vi "Kinematika.vi"() -> ()   [LabVIEW 2011]
uses:
  <vilib>/imath/engines/lvmath2/RunTimeEngine/ErrorHandling/NIMS_Finalize Error.vi
  <vilib>/imath/engines/lvmath2/RunTimeEngine/BuiltInFunctions/deg_to_rad/NIMS_deg_to_rad.vi
  <instcachedir>/0/NIMS_deg_to_rad_4A81D684CE8D4DD79924F5AB74D756E1.lvgen/NIMS_deg_to_rad_4A81D684CE8D4DD79924F5AB74D756E1_001.vi
  <vilib>/imath/engines/lvmath2/RunTimeEngine/NodeEndStatement/NIMS_NodeEndStatement_Output.vi
  <instcachedir>/0/NIMS_NodeEndStatement_Output_53EC0D466D134D7ABD903AC30B43404B.lvgen/NIMS_NodeEndStatement_Output_53EC0D466D134D7ABD903AC30B43404B_001.vi
  <instcachedir>/0/NIMS_NodeEndStatement_Output_53EC0D466D134D7ABD903AC30B43404B.lvgen/NIMS_NodeEndStatement_Output_53EC0D466D134D7ABD903AC30B43404B_012.vi
  <vilib>/imath/engines/lvmath2/RunTimeSupport/NIMS_Complex To Real.vi
  <instcachedir>/0/NIMS_Complex To Real_C6C689ECDA084B0290AC275552CC3682.lvgen/NIMS_Complex To Real_C6C689ECDA084B0290AC275552CC3682_001.vi
  <vilib>/imath/engines/lvmath2/RunTimeEngine/BuiltInFunctions/rad_to_deg/NIMS_rad_to_deg.vi
  <instcachedir>/0/NIMS_rad_to_deg_A39AFCDDC8C049FCADAAB7FC30B9F5AA.lvgen/NIMS_rad_to_deg_A39AFCDDC8C049FCADAAB7FC30B9F5AA_001.vi
  <vilib>/imathl/engines/lvmath/Functions/Error Handling/Create Error.vi
  <vilib>/imath/engines/lvmath2/RunTimeEngine/BuiltInFunctions/abs/NIMS_abs(signed).vi
  <instcachedir>/0/NIMS_abs(signed)_C4FCB8E6058B49B797C7C8D53CA5F6EC.lvgen/NIMS_abs(signed)_C4FCB8E6058B49B797C7C8D53CA5F6EC_002.vi
  <vilib>/imath/engines/lvmath2/RunTimeEngine/BuiltInFunctions/acos/NIMS_acos(C).vi
  <instcachedir>/0/NIMS_acos(C)_7CE2F6FACE8F41D2AB6320A13102A19C.lvgen/NIMS_acos(C)_7CE2F6FACE8F41D2AB6320A13102A19C_001.vi
  <vilib>/Instr/_visa.llb/VISA Configure Serial Port (Instr).vi
panel:
  in  "MOVE":bool
  in  "buffer":string
  in  "buffer":string
  out "PWM Values":T1
  in  "VISA NAME":refnum<visa-resource-name>="COM24"
  in  "STOP":bool
  in  "Dimensi Lengan Robot":cluster{"l1":dbl, "l2":dbl, "l3":dbl, "l4":dbl}={"l1"=75.0, "l2"=95.0, "l3"=95.0, "l4"=107.0} caption="Arm Dimensiions 2"
  out "TOP VIEW ROBOT":cluster{"Y":dbl[], "Y":dbl[]}[](graph)
  out "SIDE VIEW ROBOT":cluster{"Y":dbl[], "Y":dbl[]}[](graph)
  in  "Kinematik Maju / Balik":enum32{"Kinematika Maju", "Kinematika Balik"}(tab)
  out "Koordinat Akhir (KM)":cluster{"X":dbl, "Y":dbl, "Z":dbl}
  in  "BASE":dbl(knob) scale=-90.0..90.0
  in  "SHOULDER":dbl(knob)=30.0 scale=0.0..135.0
  in  "ELBOW":dbl(knob)=150.0 scale=90.0..270.0
  in  "WRIST":dbl(knob)=150.0 scale=90.0..270.0
  in  "ELBOW CONFIG":bool
  in  "Koordinat Z":dbl(slide)=75.0 scale=0.0..300.0
  in  "Koordinat Y":dbl(slide) scale=-135.0..135.0
  in  "Koordinat X":dbl(slide)=297.0 scale=0.0..300.0
  out "Sudut Persendian (KB)":cluster{"q1":dbl, "q2":dbl, "q3":dbl, "q4":dbl}
  in  "theta":dbl(knob) scale=0.0..90.0
  # "Percobaan kinematika maju ini didasarkan pada konfigurasi robot berlengan yang terintegrasi dengan sistem. \nRobot yang digunakan merupakan robot revolute yang memiliki 4 DOF ditambah satu gripper.\nRentang sudut yang diperbolehkan juga berdasarkan karakteristik penggerak robot\n\nParameter D-H  robot dapat dilihat pada tabel disamping."
  # "Percobaan kinematika balik ini merupakan perhitungan balik dari \npercobaan kinematika maju pada tab sebelumnya.\nsolusi kinematika balik yang beragam ditampilkan pada simulasi\ndengan memilih konfigurasi elbow up atau elbow down \nnamun robot berlengan yang terintegrasi dengan sistem hanya \nmenggunakan konfigurasi elbow up"
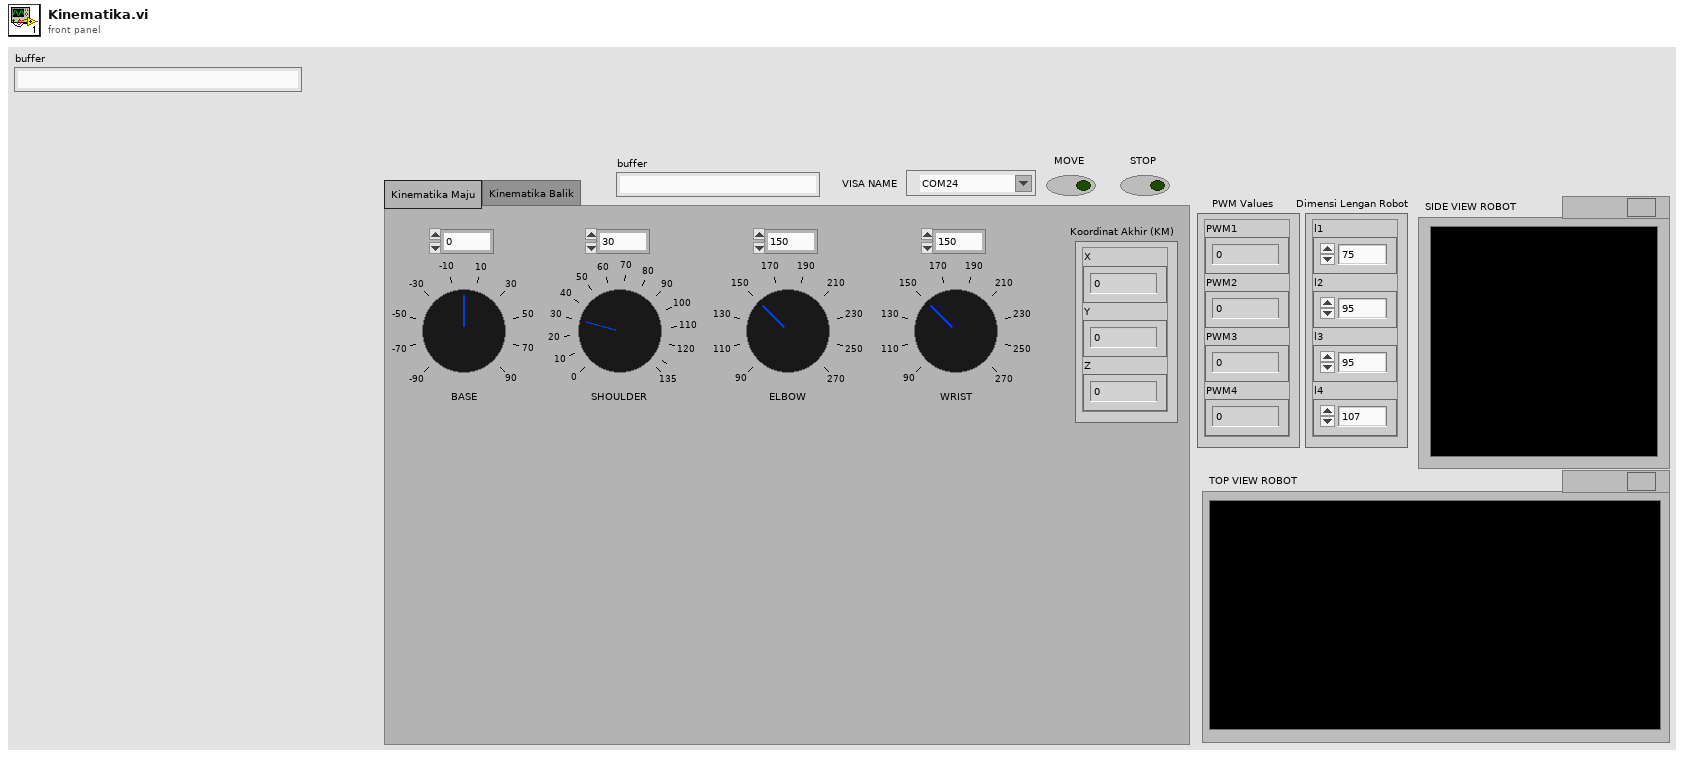
[diagram p1: front panel]
types:
  T1 = cluster{"PWM1":u32, "PWM2":u32, "PWM3":u32, "PWM4":u32}
  T2 = cluster{"PW1":u32, "PW2":u32, "PW3":u32, "PW4":u32}
  T3 = cluster{"Theta0":dbl, "Theta1":dbl, "Theta2":dbl}
  T4 = cluster{"Theta0":dbl, "Theta1":dbl, "Theta2":dbl, "Theta3":dbl}
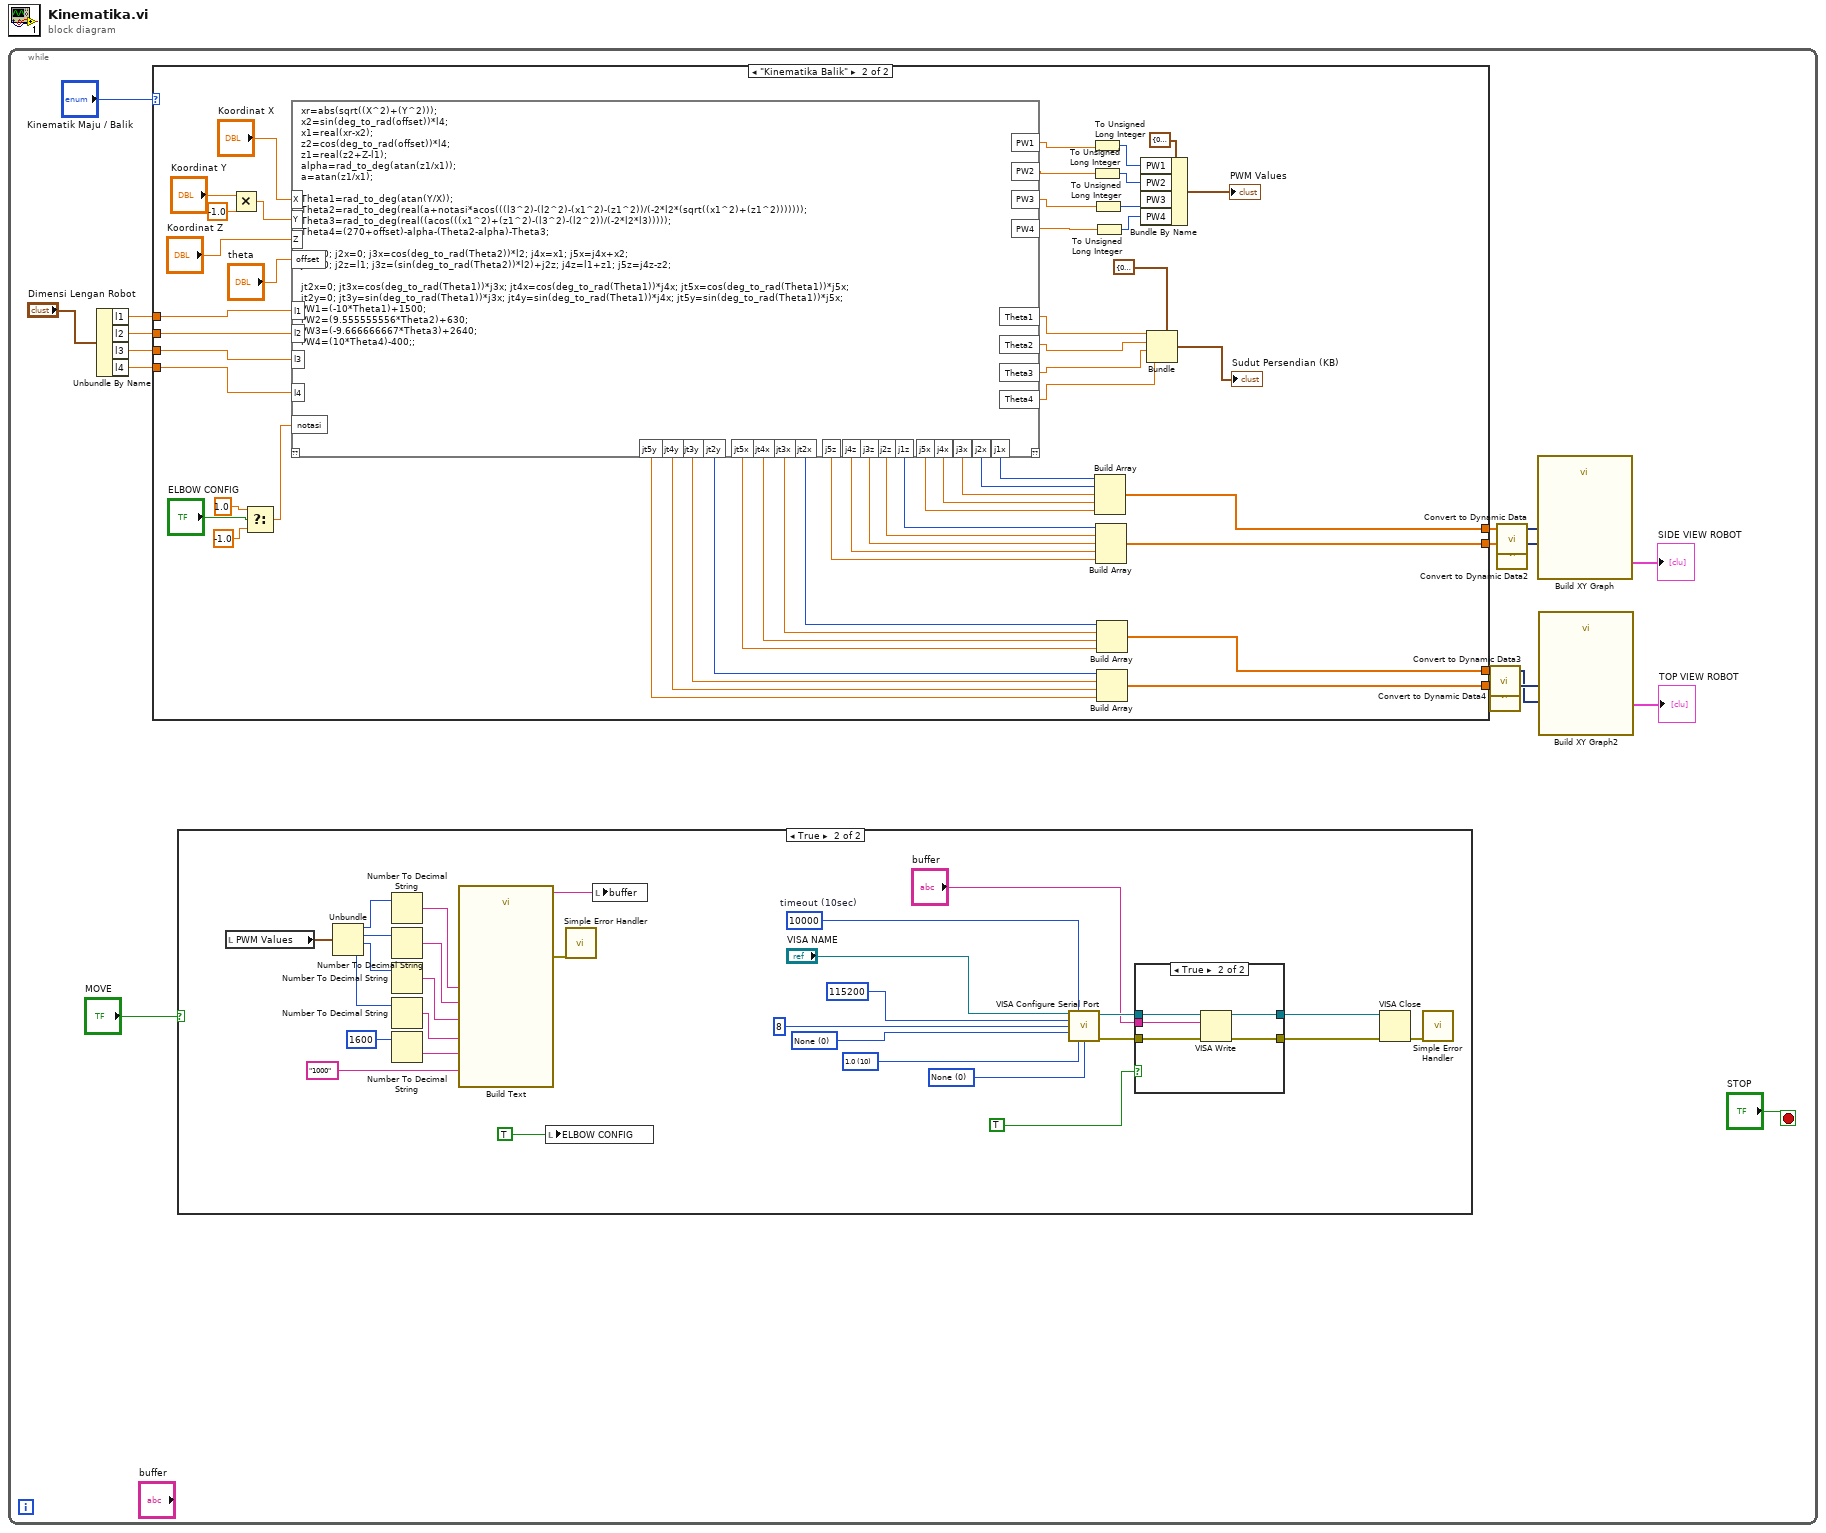
[diagram p0: block diagram]
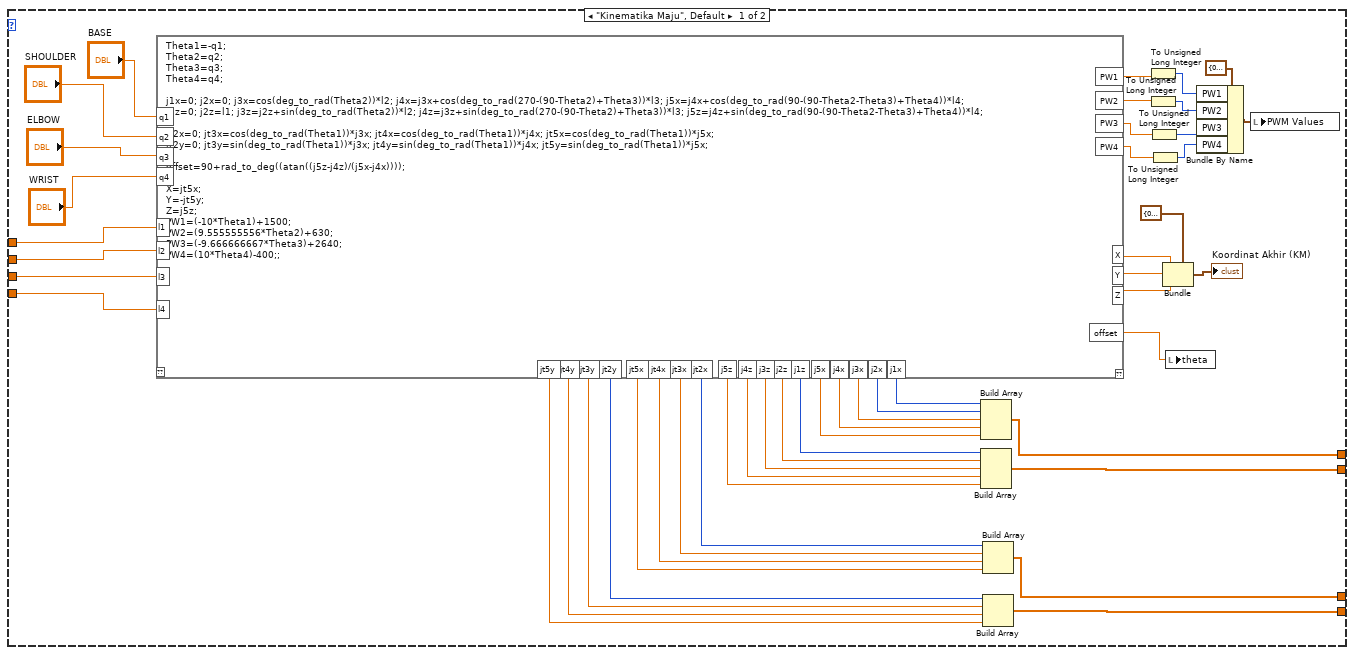
[diagram p4: hidden frame]
diagram:
  n1 = while {
    stop <- "STOP" stop-if-true
    n2 = Unbundle By Name("Dimensi Lengan Robot") -> ("l1"=w7:dbl, "l2"=w6:dbl, "l3"=w5:dbl, "l4"=w4:dbl)
    n3 = case shown="\"Kinematika Balik\"" "Kinematik Maju / Balik" {
      tunnel: [w100 w498] -> w12
      tunnel: [w99 w497] -> w11
      tunnel: [w98 w496] -> w10
      tunnel: [w97 w495] -> w9
      tunnel: w7 -> [w96 w494]
      tunnel: w6 -> [w95 w493]
      tunnel: w5 -> [w94 w492]
      tunnel: w4 -> [w93 w491]
      frame "Kinematika Maju", Default {
        n4 = mathscript code="Theta1=-q1;\nTheta2=q2;\nTheta3=q3;\nTheta4=q4;\n\nj1x=0; j2x=0; j3x=cos(deg_to_rad(Theta2))*l2; j4x=j3x+cos(deg_to_rad(270-(90-Theta2)+Theta3))*l3; j5x=j4x+cos(deg_to_rad(90-(90-Theta2-Theta3)+Theta4))*l4;\nj1z=0; j2z=l1; j3z=j2z+sin(deg_to_rad(Theta2))*l2; j4z=j3z+sin(deg_to_rad(270-(90-Theta2)+Theta3))*l3; j5z=j4z+sin(deg_to_rad(90-(90-Theta2-Theta3)+Theta4))*l4;\n\njt2x=0; jt3x=cos(deg_to_rad(Theta1))*j3x; jt4x=cos(deg_to_rad(Theta1))*j4x; jt5x=cos(deg_to_rad(Theta1))*j5x;\njt2y=0; jt3y=sin(deg_to_rad(Theta1))*j3x; jt4y=sin(deg_to_rad(Theta1))*j4x; jt5y=sin(deg_to_rad(Theta1))*j5x;\n\noffset=90+rad_to_deg((atan((j5z-j4z)/(j5x-j4x))));\n\nX=jt5x;\nY=-jt5y;\nZ=j5z;\nPW1=(-10*Theta1)+1500;\nPW2=(9.555555556*Theta2)+630;\nPW3=(-9.666666667*Theta3)+2640;\nPW4=(10*Theta4)-400;;"("q1"="BASE", "q2"="SHOULDER", "q3"="ELBOW", "l2"=w95, "l3"=w94, "l4"=w93, "l1"=w96, "q4"="WRIST") -> ("j1x"=w82:i32, "j2x"=w81:i32, "j3x"=w80:dbl, "j4x"=w79:dbl, "j1z"=w77:i32, "j2z"=w76:dbl, "j3z"=w75:dbl, "j4z"=w74:dbl, "jt2x"=w72:i32, "jt3x"=w71:dbl, "jt4x"=w70:dbl, "jt2y"=w68:i32, "jt3y"=w67:dbl, "jt4y"=w66:dbl, "X"=w92:dbl, "Y"=w91:dbl, "Z"=w90:dbl, "offset"=w83:dbl, "j5x"=w78:dbl, "j5z"=w73:dbl, "jt5x"=w69:dbl, "jt5y"=w65:dbl, "PW1"=w59:dbl, "PW2"=w58:dbl, "PW3"=w57:dbl, "PW4"=w56:dbl)  [unwired: 1 in, 1 out]
        n5 = Build Array(w82, w81, w80, w79, w78) -> (w100:dbl[])
        n6 = Build Array(w77, w76, w75, w74, w73) -> (w99:dbl[])
        n7 = Build Array(w72, w71, w70, w69) -> (w98:dbl[])
        n8 = Build Array(w68, w67, w66, w65) -> (w97:dbl[])
        n9 = To Unsigned Long Integer(number=w59) -> (unsigned 32bit integer=w64:u32)
        n10 = To Unsigned Long Integer(number=w58) -> (unsigned 32bit integer=w62:u32)
        n11 = To Unsigned Long Integer(number=w57) -> (unsigned 32bit integer=w61:u32)
        n12 = To Unsigned Long Integer(number=w56) -> (unsigned 32bit integer=w60:u32)
        n13 = Bundle(cluster=T3 {"Theta0"=0.0, "Theta1"=0.0, "Theta2"=0.0} ("Joint Angles"), "Theta0"=w92, "Theta1"=w91, "Theta2"=w90) -> (→"Koordinat Akhir (KM)":T3)
        n14 = local write "theta"(w83) -> ()
        n15 = Bundle By Name(cluster=T2 {"PW1"=0, "PW2"=0, "PW3"=0, "PW4"=0} ("PWM Values 2"), "PW1"=w64, "PW2"=w62, "PW3"=w61, "PW4"=w60) -> (w55:T2)
        n16 = local write "PWM Values"(w55) -> ()
      }
      frame "Kinematika Balik" {
        # "Enter constants for your servo calibrations here"
        n17 = Multiply(x="Koordinat Y", y=-1.0) -> (x*y=w486:dbl)
        n18 = Select(t=1.0, s="ELBOW CONFIG", f=-1.0) -> (s? t:f=w457:dbl)
        n19 = mathscript code="xr=abs(sqrt((X^2)+(Y^2)));\nx2=sin(deg_to_rad(offset))*l4;\nx1=real(xr-x2);\nz2=cos(deg_to_rad(offset))*l4;\nz1=real(z2+Z-l1);\nalpha=rad_to_deg(atan(z1/x1));\na=atan(z1/x1);\n\nTheta1=rad_to_deg(atan(Y/X));\nTheta2=rad_to_deg(real(a+notasi*acos(((l3^2)-(l2^2)-(x1^2)-(z1^2))/(-2*l2*(sqrt((x1^2)+(z1^2)))))));\nTheta3=rad_to_deg(real((acos(((x1^2)+(z1^2)-(l3^2)-(l2^2))/(-2*l2*l3)))));\nTheta4=(270+offset)-alpha-(Theta2-alpha)-Theta3;\n\nj1x=0; j2x=0; j3x=cos(deg_to_rad(Theta2))*l2; j4x=x1; j5x=j4x+x2;\nj1z=0; j2z=l1; j3z=(sin(deg_to_rad(Theta2))*l2)+j2z; j4z=l1+z1; j5z=j4z-z2;\n\njt2x=0; jt3x=cos(deg_to_rad(Theta1))*j3x; jt4x=cos(deg_to_rad(Theta1))*j4x; jt5x=cos(deg_to_rad(Theta1))*j5x;\njt2y=0; jt3y=sin(deg_to_rad(Theta1))*j3x; jt4y=sin(deg_to_rad(Theta1))*j4x; jt5y=sin(deg_to_rad(Theta1))*j5x;\nPW1=(-10*Theta1)+1500;\nPW2=(9.555555556*Theta2)+630;\nPW3=(-9.666666667*Theta3)+2640;\nPW4=(10*Theta4)-400;;"("X"="Koordinat X", "Y"=w486, "Z"="Koordinat Z", "l2"=w493, "l3"=w492, "l4"=w491, "l1"=w494, "offset"="theta", "notasi"=w457) -> ("Theta1"=w484:dbl, "Theta2"=w483:dbl, "Theta3"=w482:dbl, "j1x"=w478:i32, "j2x"=w477:i32, "j3x"=w476:dbl, "j4x"=w475:dbl, "j1z"=w473:i32, "j2z"=w472:dbl, "j3z"=w471:dbl, "j4z"=w470:dbl, "jt2x"=w468:i32, "jt3x"=w467:dbl, "jt4x"=w466:dbl, "jt2y"=w464:i32, "jt3y"=w463:dbl, "jt4y"=w462:dbl, "Theta4"=w481:dbl, "j5x"=w474:dbl, "j5z"=w469:dbl, "jt5x"=w465:dbl, "jt5y"=w461:dbl, "PW1"=w447:dbl, "PW2"=w448:dbl, "PW3"=w449:dbl, "PW4"=w450:dbl)  [unwired: 1 in, 1 out]
        n20 = To Unsigned Long Integer(number=w447) -> (unsigned 32bit integer=w456:u32)
        n21 = To Unsigned Long Integer(number=w448) -> (unsigned 32bit integer=w454:u32)
        n22 = To Unsigned Long Integer(number=w449) -> (unsigned 32bit integer=w453:u32)
        n23 = To Unsigned Long Integer(number=w450) -> (unsigned 32bit integer=w452:u32)
        n24 = Build Array(w478, w477, w476, w475, w474) -> (w498:dbl[])
        n25 = Build Array(w473, w472, w471, w470, w469) -> (w497:dbl[])
        n26 = Build Array(w468, w467, w466, w465) -> (w496:dbl[])
        n27 = Build Array(w464, w463, w462, w461) -> (w495:dbl[])
        n28 = Bundle By Name(cluster=T2 {"PW1"=0, "PW2"=0, "PW3"=0, "PW4"=0} ("PWM Values 2"), "PW1"=w456, "PW2"=w454, "PW3"=w453, "PW4"=w452) -> (→"PWM Values":T2)
        n29 = Bundle(cluster=T4 {"Theta0"=0.0, "Theta1"=0.0, "Theta2"=0.0, "Theta3"=0.0} ("Joint Angles"), "Theta0"=w484, "Theta1"=w483, "Theta2"=w482, "Theta3"=w481) -> (→"Sudut Persendian (KB)":T4)
      }
    }
    n30 = case shown="True" "MOVE" {
      frame False {
      }
      frame True {
        w41 = u16 0 items=["None"=0, "XON/XOFF"=1, "RTS/CTS"=2, "DTR/DSR"=4] ("flow control")
        w42 = u16 10 items=["1.0"=10, "1.5"=15, "2.0"=20] ("stop bits")
        w44 = u16 0 items=["None", "Odd", "Even", "Mark", "Space"] ("parity")
        w43 = u32 10000  # timeout (10sec)
        n31 = local read "PWM Values"() -> (w26:T1)
        n32 = Unbundle(w26) -> ("PWM1"=w31:u32, "PWM2"=w32:u32, "PWM3"=w33:u32, "PWM4"=w34:u32)
        n33 = Number To Decimal String(number=w31) -> (decimal integer string=w25:string)  [unwired: 1 in]
        n34 = Number To Decimal String(number=w32) -> (decimal integer string=w27:string)  [unwired: 1 in]
        n35 = Number To Decimal String(number=w33) -> (decimal integer string=w28:string)  [unwired: 1 in]
        n36 = Number To Decimal String(number=w34) -> (decimal integer string=w29:string)  [unwired: 1 in]
        n37 = Number To Decimal String(number=1600) -> (decimal integer string=w30:string)  [unwired: 1 in]
        n38 = call "Build Text"("pwm3"=w29, "time"="1000", "pwm0"=w25, "pwm1"=w27, "pwm2"=w28, "pwm4"=w30) -> ("Result"=w20:string, "error out"=w24:errorcluster)  [unwired: 8 in]
        n39 = local write "ELBOW CONFIG"(TRUE ("ELBOW CONFIG")) -> ()
        n40 = call <vilib>:"Simple Error Handler.vi"("error in (no error)"=w24) -> ()  [unwired: 4 in, 5 out]
        n41 = local write "buffer"(w20) -> ()
        n42 = call-poly "VISA Configure Serial Port"("VISA resource name"="VISA NAME", "timeout (10sec)"=w43, "baud rate (9600)"=u32 115200 ("baud rate"), "data bits (8)"=u16 8 ("data bits"), "parity (0:none)"=w44, "stop bits (10: 1 bit)"=w42, "flow control (0:none)"=w41) -> ("VISA resource name out"=w39:refnum<visa-resource-name>, "error out"=w38:errorcluster)  [unwired: 7 in]
        n43 = case shown="True" TRUE ("WRITE") {
          tunnel: w39 -> [w49 w54]
          tunnel: w38 -> [w48 w53]
          tunnel: [w49 w52] -> w36
          tunnel: [w48 w51] -> w35
          tunnel: "buffer" -> [_ w50]
          frame False {
          }
          frame True {
            n44 = VISA Write(VISA resource name=w54, write buffer=w50, error in (no error)=w53) -> (VISA resource name out=w52:refnum<visa-resource-name>, error out=w51:errorcluster)  [unwired: 1 out]
          }
        }
        n45 = VISA Close(VISA resource name=w36, error in (no error)=w35) -> (error out=w45:errorcluster)
        n46 = call <vilib>:"Simple Error Handler.vi"("error in (no error)"=w45) -> ()  [unwired: 4 in, 5 out]
      }
    }
    n47 = call "Convert to Dynamic Data3"("Array"=w10) -> ("Dynamic Data Type"=w13:dynamicdata)  [unwired: 3 in]
    n48 = call "Convert to Dynamic Data4"("Array"=w9) -> ("Dynamic Data Type"=w14:dynamicdata)  [unwired: 3 in]
    n49 = call "Convert to Dynamic Data"("Array"=w12) -> ("Dynamic Data Type"=w17:dynamicdata)  [unwired: 3 in]
    n50 = call "Convert to Dynamic Data2"("Array"=w11) -> ("Dynamic Data Type"=w16:dynamicdata)  [unwired: 3 in]
    n51 = call "Build XY Graph"("Y Input"=w16, "X Input"=w17) -> ("XY Graph"=→"SIDE VIEW ROBOT":cluster{"Y":dbl[], "Y":dbl[]}[])  [unwired: 3 in, 6 out]
    n52 = call "Build XY Graph2"("Y Input"=w13, "X Input"=w14) -> ("XY Graph"=→"TOP VIEW ROBOT":cluster{"Y":dbl[], "Y":dbl[]}[])  [unwired: 3 in, 6 out]
  }
